vi "SerialPort.Query.vi"(6 "Wait_ms":u32=10, 7 "TimeOut":u32=100 caption="TimeOut_ms", 8 "error in (no error)":errorcluster, 9 "Term Str":string, 10 "Cmd":string, 11 "SerialPort in":refnum<class "SerialPort.lvclass">) -> (0 "error out":errorcluster, 1 "Response":string, 2 "Made Connection":bool, 3 "SerialPort out":refnum<class "SerialPort.lvclass">, 4 "Dur_ms":u32=10)   [LabVIEW 2018, in "SerialPort.lvclass"]
uses:
  SerialPort.lvclass
  SerialPort.lvclass/SerialPort.ctl
  Utils/Errors/Error.Error Code List.ctl
  Controls/SerialPort.Status Enum.ctl
panel:
  out "Start":u32
  # "Send Cmd\nRead until either TimeOut or Term String recieved"
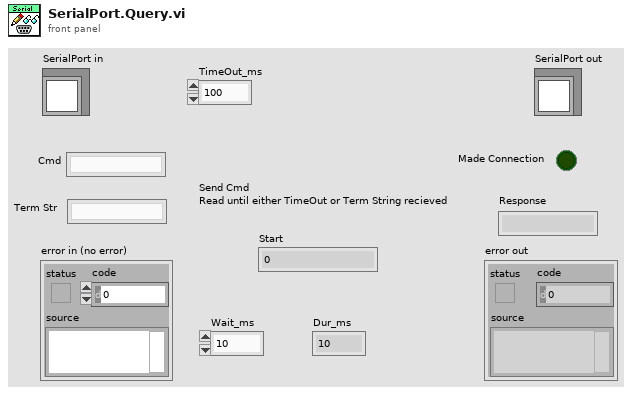
[diagram p1: front panel]
types:
  T1 = typedef "SerialPort.Status Enum.ctl" = enum16{"Disconnected", "Connecting", "Connected"}
  T2 = typedef "Error.Error Code List.ctl" = i32
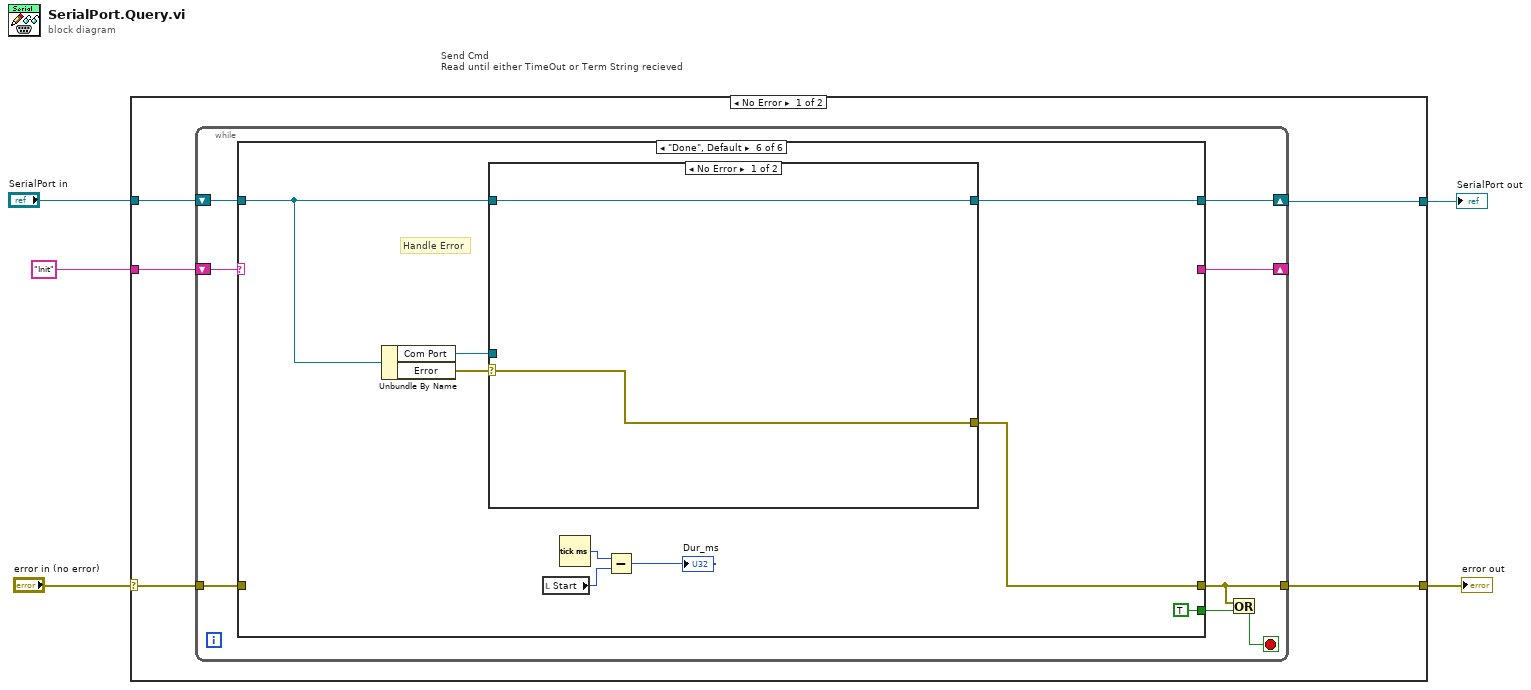
[diagram p0: block diagram]
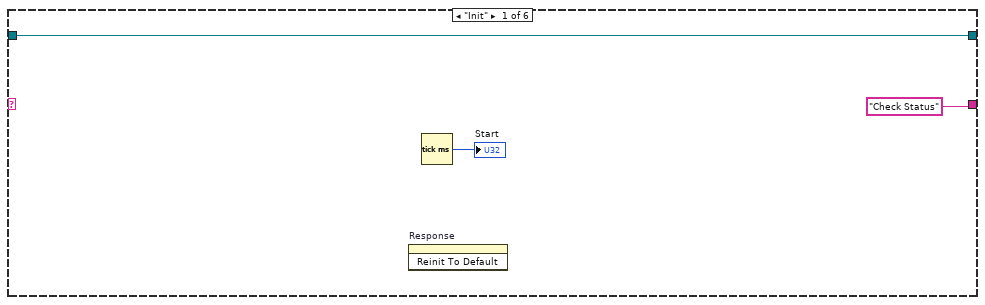
[diagram p2: hidden frame]
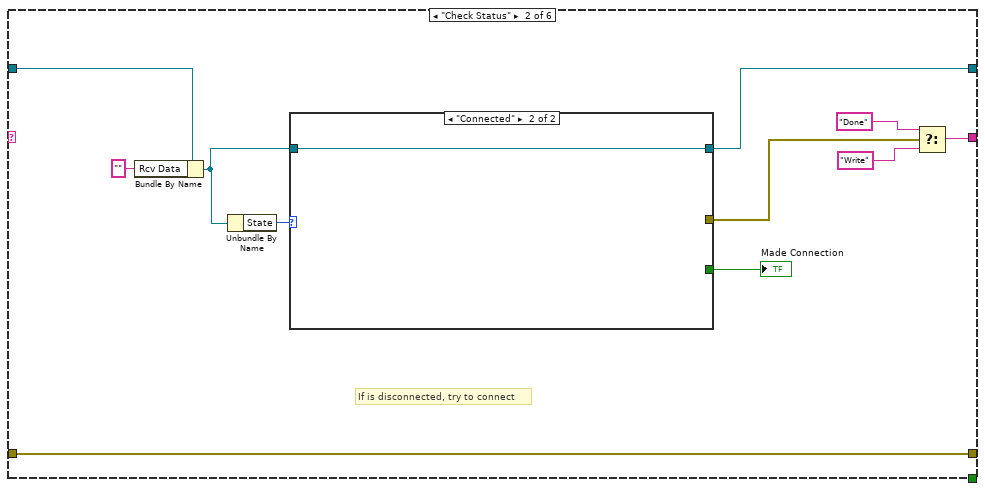
[diagram p3: hidden frame]
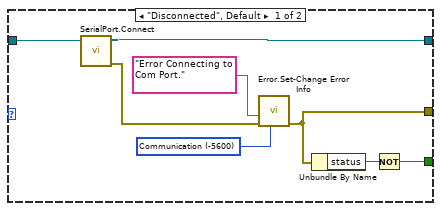
[diagram p4: hidden frame]
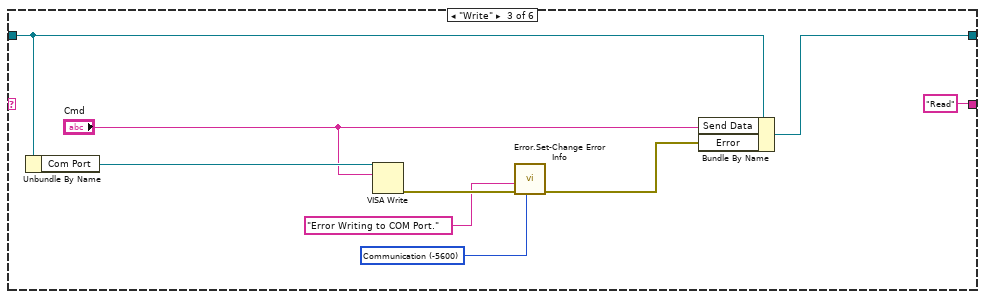
[diagram p5: hidden frame]
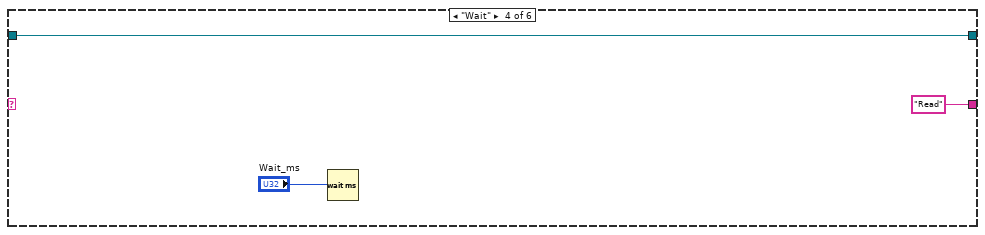
[diagram p6: hidden frame]
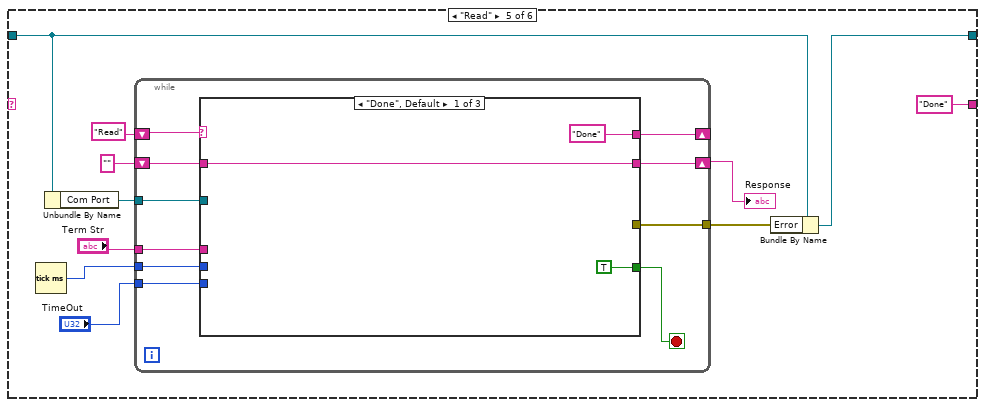
[diagram p7: hidden frame]
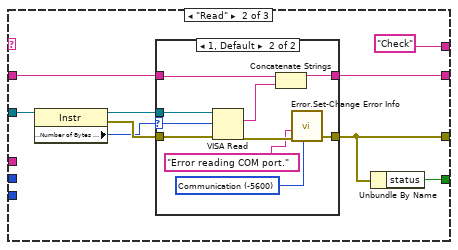
[diagram p8: hidden frame]
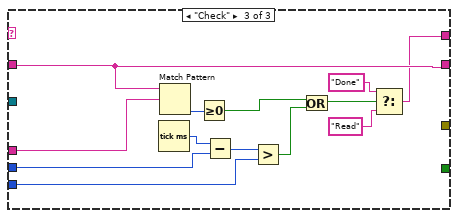
[diagram p10: hidden frame]
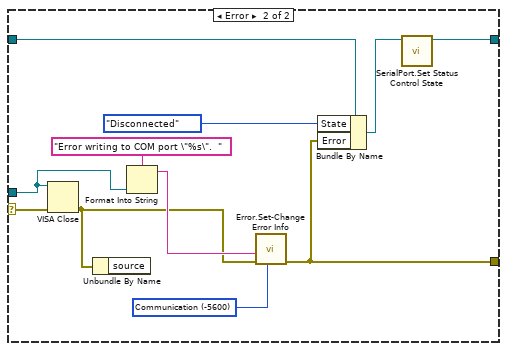
[diagram p11: hidden frame]
diagram:
  # "Send Cmd\nRead until either TimeOut or Term String recieved"
  n1 = case shown="No Error" "error in (no error)" {
    selector: "error in (no error)" -> [w6 w134]
    tunnel: [w8 w134] -> w4
    tunnel: [w7 w133] -> w2
    tunnel: "SerialPort in" -> [w10 w133]
    tunnel: "Init" -> [w9 _]
    frame No Error {
      n2 = while {
        shift-right: [w16] -> w7
        shift-left: w10 -> [w17]
        shift-right: [w15] -> _
        shift-left: w9 -> [w18]
        tunnel: [w14] -> w8
        tunnel: w6 -> [w11]
        stop <- w12 stop-if-true
        n3 = case shown="\"Done\", Default" w18 {
          tunnel: w17 -> [w21 w26 w49 w52 w61 w119]
          tunnel: [w21 w31 w48 w52 w62 w115] -> w16
          tunnel: ["Check Status" w30 "Read" "Read" "Done" _] -> w15
          tunnel: [_ w23 _ _ _ w117] -> w14
          tunnel: [_ _ _ _ _ TRUE] -> w13
          tunnel: w11 -> [_ w23 _ _ _ _]
          frame "Init" {
            n4 = invoke on="Response" class="Str" method="Reinit To Default"() -> ()  [unwired: 3 in, 3 out]
            n5 = Tick Count (ms)() -> (millisecond timer value=→"Start":u32)
          }
          frame "Check Status" {
            # "If is disconnected, try to connect"
            n6 = Bundle By Name(cluster=w26, "Rcv Data"="") -> (w25:refnum<class "SerialPort.lvclass">)
            n7 = Unbundle By Name(w25) -> ("State"=w32:T1)
            n8 = case shown="\"Connected\"" w32 {
              tunnel: w25 -> [w40 w41]
              tunnel: [w39 w41] -> w31
              tunnel: [w35 _] -> w29
              tunnel: [w37 _] -> w22
              frame "Disconnected", Default {
                w33 = T2 -5600 items=["No Error"=0, "Abort"=-2, "Misc"=-5000, "Fixture Error"=-5100, "File IO - General"=-5200, "FIle IO - Config Error"=-5201, "Instrument - General"=-5300, "Instrument - Serial Com"=-5301, "Instrument - Camera"=-5302, "Instrument - PS"=-5303, "Instrument - Oscilloscope"=-5304, "Instrument - Function Gen"=-5305, "Instrument - Load"=-5306, "Instrument - Meter"=-5307, "Instrument - Power Control"=-5308, "Instrument - Motion"=-5309, "Instrument - RF"=-5310, "System Exe"=-5400, "Image Processing"=-5500, "Communication"=-5600, "Script - Syntax Error"=-6000, "Script - Invalid Name or Param"=-6100, "Script - Timeout"=-6200, "Invalid Data"=-6300] ("Std Code")
                n9 = call "SerialPort.Connect.vi"("SerialPort in"=w40) -> ("error out"=w36:errorcluster, "SerialPort out"=w39:refnum<class "SerialPort.lvclass">)  [unwired: 8 in, 1 out]
                n10 = call "Error.Set-Change Error Info.vi"("Std Code"=w33, "error in"=w36, "Description"="Error Connecting to Com Port.") -> ("error out"=w35:errorcluster)  [unwired: 8 in]
                n11 = Unbundle By Name(w35) -> ("status"=w38:bool)
                n12 = Not(x=w38) -> (.not. x?=w37:bool)
              }
              frame "Connected" {
              }
            }
            "Made Connection" <- w22
            n13 = Select(t="Done", s=w29, f="Write") -> (s? t:f=w30:string)
          }
          frame "Write" {
            w43 = T2 -5600 items=["No Error"=0, "Abort"=-2, "Misc"=-5000, "Fixture Error"=-5100, "File IO - General"=-5200, "FIle IO - Config Error"=-5201, "Instrument - General"=-5300, "Instrument - Serial Com"=-5301, "Instrument - Camera"=-5302, "Instrument - PS"=-5303, "Instrument - Oscilloscope"=-5304, "Instrument - Function Gen"=-5305, "Instrument - Load"=-5306, "Instrument - Meter"=-5307, "Instrument - Power Control"=-5308, "Instrument - Motion"=-5309, "Instrument - RF"=-5310, "System Exe"=-5400, "Image Processing"=-5500, "Communication"=-5600, "Script - Syntax Error"=-6000, "Script - Invalid Name or Param"=-6100, "Script - Timeout"=-6200, "Invalid Data"=-6300] ("Std Code")
            n14 = Unbundle By Name(w49) -> ("Com Port"=w47:refnum<visa-resource-name>)
            n15 = VISA Write(VISA resource name=w47, write buffer="Cmd") -> (error out=w45:errorcluster)  [unwired: 1 in, 2 out]
            n16 = call "Error.Set-Change Error Info.vi"("Std Code"=w43, "error in"=w45, "Description"="Error Writing to COM Port.") -> ("error out"=w42:errorcluster)  [unwired: 8 in]
            n17 = Bundle By Name(cluster=w49, "Send Data"="Cmd", "Error"=w42) -> (w48:refnum<class "SerialPort.lvclass">)
          }
          frame "Wait" {
            n18 = Wait (ms)(milliseconds to wait="Wait_ms") -> ()  [unwired: 1 out]
          }
          frame "Read" {
            n19 = Tick Count (ms)() -> (millisecond timer value=w55:u32)
            n20 = Unbundle By Name(w61) -> ("Com Port"=w64:refnum<visa-resource-name>)
            n21 = while {
              tunnel: w64 -> [w74]
              tunnel: [w73] -> w59
              shift-right: [w71] -> w57
              shift-left: "" -> [w72]
              tunnel: w55 -> [w66]
              tunnel: "TimeOut" -> [w65]
              shift-right: [w69] -> _
              shift-left: "Read" -> [w70]
              tunnel: "Term Str" -> [w67]
              stop <- w68 stop-if-true
              n22 = case shown="\"Done\", Default" w70 {
                tunnel: w74 -> [_ w85 _]
                tunnel: [_ w79 _] -> w73
                tunnel: w72 -> [w77 w82 w104]
                tunnel: [w77 w81 w104] -> w71
                tunnel: ["Done" "Check" w101] -> w69
                tunnel: [TRUE w78 _] -> w68
                tunnel: w67 -> [_ _ w111]
                tunnel: w66 -> [_ _ w108]
                tunnel: w65 -> [_ _ w107]
                frame "Done", Default {
                }
                frame "Read" {
                  n23 = property class="Instr"(reference=w85) -> (reference out=w86:refnum<visa-resource-name>, error out=w84:errorcluster, "Serial Settings:Number of Bytes at Serial Port"=w83:u32)  [unwired: 1 in]
                  n24 = case shown="1, Default" w83 {
                    selector: w83 -> [_ w96]
                    tunnel: w86 -> [_ w98]
                    tunnel: w84 -> [w88 w97]
                    tunnel: [w88 w92] -> w79
                    tunnel: w82 -> [w87 w94]
                    tunnel: [w87 w95] -> w81
                    frame 0 {
                    }
                    frame 1, Default {
                      w90 = T2 -5600 items=["No Error"=0, "Abort"=-2, "Misc"=-5000, "Fixture Error"=-5100, "File IO - General"=-5200, "FIle IO - Config Error"=-5201, "Instrument - General"=-5300, "Instrument - Serial Com"=-5301, "Instrument - Camera"=-5302, "Instrument - PS"=-5303, "Instrument - Oscilloscope"=-5304, "Instrument - Function Gen"=-5305, "Instrument - Load"=-5306, "Instrument - Meter"=-5307, "Instrument - Power Control"=-5308, "Instrument - Motion"=-5309, "Instrument - RF"=-5310, "System Exe"=-5400, "Image Processing"=-5500, "Communication"=-5600, "Script - Syntax Error"=-6000, "Script - Invalid Name or Param"=-6100, "Script - Timeout"=-6200, "Invalid Data"=-6300] ("Std Code")
                      n25 = VISA Read(VISA resource name=w98, byte count=w96, error in (no error)=w97) -> (read buffer=w93:string, error out=w91:errorcluster)  [unwired: 2 out]
                      n26 = Concatenate Strings(w94, w93) -> (w95:string)
                      n27 = call "Error.Set-Change Error Info.vi"("Std Code"=w90, "error in"=w91, "Description"="Error reading COM port.") -> ("error out"=w92:errorcluster)  [unwired: 8 in]
                    }
                  }
                  n28 = Unbundle By Name(w79) -> ("status"=w78:bool)
                }
                frame "Check" {
                  n29 = Tick Count (ms)() -> (millisecond timer value=w109:u32)
                  n30 = Match Pattern(string=w104, regular expression=w111) -> (offset past match=w110:i32)  [unwired: 1 in, 3 out]
                  n31 = Greater Or Equal To 0?(x=w110) -> (x >= 0?=w105:bool)
                  n32 = Subtract(x=w109, y=w108) -> (x-y=w99:u32)
                  n33 = Greater?(x=w99, y=w107) -> (0:w106:bool)
                  n34 = Or(x=w105, y=w106) -> (x .or. y?=w100:bool)
                  n35 = Select(t="Done", s=w100, f="Read") -> (s? t:f=w101:string)
                }
              }
            }
            "Response" <- w57
            n36 = Bundle By Name(cluster=w61, "Error"=w59) -> (w62:refnum<class "SerialPort.lvclass">)
          }
          frame "Done", Default {
            # "Handle Error"
            n37 = Unbundle By Name(w119) -> ("Com Port"=w118:refnum<visa-resource-name>, "Error"=w120:errorcluster)
            n38 = case shown="No Error" w120 {
              selector: w120 -> [w122 w124]
              tunnel: w119 -> [w121 w130]
              tunnel: [w121 w128] -> w115
              tunnel: w118 -> [_ w129]
              tunnel: [w122 w126] -> w117
              frame No Error {
              }
              frame Error {
                w123 = T2 -5600 items=["No Error"=0, "Abort"=-2, "Misc"=-5000, "Fixture Error"=-5100, "File IO - General"=-5200, "FIle IO - Config Error"=-5201, "Instrument - General"=-5300, "Instrument - Serial Com"=-5301, "Instrument - Camera"=-5302, "Instrument - PS"=-5303, "Instrument - Oscilloscope"=-5304, "Instrument - Function Gen"=-5305, "Instrument - Load"=-5306, "Instrument - Meter"=-5307, "Instrument - Power Control"=-5308, "Instrument - Motion"=-5309, "Instrument - RF"=-5310, "System Exe"=-5400, "Image Processing"=-5500, "Communication"=-5600, "Script - Syntax Error"=-6000, "Script - Invalid Name or Param"=-6100, "Script - Timeout"=-6200, "Invalid Data"=-6300] ("Std Code")
                n39 = VISA Close(VISA resource name=w129) -> ()  [unwired: 1 in, 1 out]
                n40 = Unbundle By Name(w124) -> ()  [unwired: 1 out]
                n41 = Format Into String(format string="Error writing to COM port \"%s\".  ", w129) -> (resulting string=w125:string)  [unwired: 2 in, 1 out]
                n42 = call "Error.Set-Change Error Info.vi"("Std Code"=w123, "error in"=w124, "Description"=w125) -> ("error out"=w126:errorcluster)  [unwired: 8 in]
                n43 = Bundle By Name(cluster=w130, "State"=SerialPort.Status_Enum."Disconnected", "Error"=w126) -> (w127:refnum<class "SerialPort.lvclass">)
                n44 = call "SerialPort.Set Status Control State.vi"("SerialPort in"=w127) -> ("SerialPort out"=w128:refnum<class "SerialPort.lvclass">)  [unwired: 9 in, 1 out]
              }
            }
            n45 = local read "Start"() -> (w113:u32)
            n46 = Tick Count (ms)() -> (millisecond timer value=w114:u32)
            n47 = Subtract(x=w114, y=w113) -> (x-y=→"Dur_ms":u32)
          }
        }
        n48 = Or(x=w14, y=w13) -> (x .or. y?=w12:bool)
      }
    }
    frame Error {
    }
  }
  "error out" <- w4
  "SerialPort out" <- w2
